vi "Proc TXed.vi"(6 "counter in":i32, 7 "Send":bool, 8 "error in":errorcluster, 9 "MsgBox in":string, 10 "Nickname":string, 11 "Connection in":refnum<k5>) -> (0 "error out":errorcluster, 1 "MsgBox out":string, 3 "Connection out":refnum<k5>, 4 "counter out":i32)   [LabVIEW 2012]
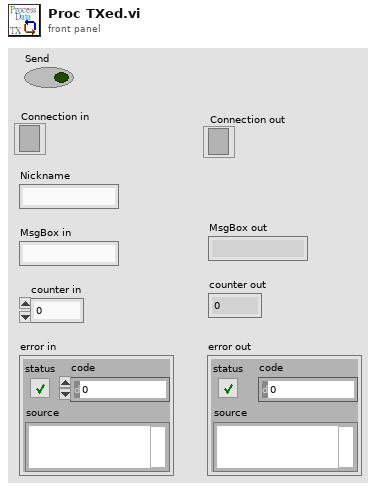
[diagram p1: front panel]
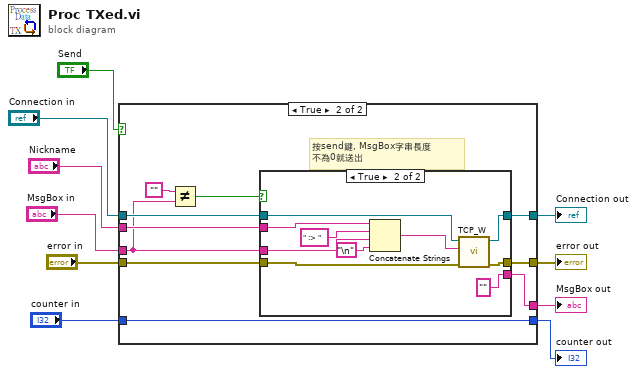
[diagram p0: block diagram]
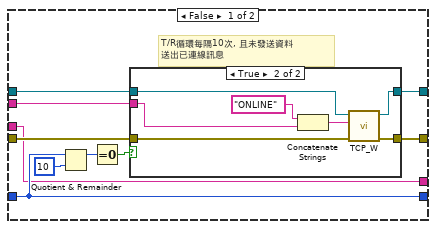
[diagram p2: hidden frame]
diagram:
  n1 = case shown="True" "Send" {
    tunnel: "Connection in" -> [w20 w38]
    tunnel: [w19 w37] -> w2
    tunnel: "error in" -> [w18 w39]
    tunnel: [w17 w36] -> w7
    tunnel: "counter in" -> [w13 w35]
    tunnel: [w13 w35] -> w5
    tunnel: "MsgBox in" -> [w12 w31]
    tunnel: [w12 w34] -> w8
    tunnel: "Nickname" -> [w11 w33]
    frame False {
      # "T/R循環每隔10次, 且未發送資料\n送出已連線訊息"
      n2 = Quotient & Remainder(x=w13, y=10) -> (x-y*floor(x/y)=w16:i32)  [unwired: 1 out]
      n3 = Equal To 0?(x=w16) -> (x = 0?=w14:bool)
      n4 = case shown="True" w14 {
        tunnel: w20 -> [w21 w29]
        tunnel: [w21 w28] -> w19
        tunnel: w18 -> [w22 w23]
        tunnel: [w22 w27] -> w17
        tunnel: w11 -> [_ w24]
        frame False {
        }
        frame True {
          n5 = Concatenate Strings("ONLINE" ("data in"), w24) -> (w25:string)
          n6 = call "TCP_W.vi"("error in"=w23, "data in"=w25, "connection ID"=w29) -> ("error IO"=w27:errorcluster, "connection ID out"=w28:refnum<k5>)  [unwired: 7 in]
        }
      }
    }
    frame True {
      # "按send鍵, MsgBox字串長度\n不為0就送出"
      n7 = Not Equal?(x="", y=w31) -> (x != y?=w32:bool)
      n8 = case shown="True" w32 {
        tunnel: w38 -> [w41 w49]
        tunnel: w39 -> [w42 w44]
        tunnel: [w42 w45] -> w36
        tunnel: w31 -> [w40 w48]
        tunnel: [w41 w47] -> w37
        tunnel: [w40 "" ("MsgBox")] -> w34
        tunnel: w33 -> [_ w43]
        frame False {
        }
        frame True {
          n9 = Concatenate Strings(w43, " :> ", w48, "\n") -> (w50:string)
          n10 = call "TCP_W.vi"("error in"=w44, "data in"=w50, "connection ID"=w49) -> ("error IO"=w45:errorcluster, "connection ID out"=w47:refnum<k5>)  [unwired: 7 in]
        }
      }
    }
  }
  "MsgBox out" <- w8
  "error out" <- w7
  "counter out" <- w5
  "Connection out" <- w2
